vi "niFpgaHandshakeEmulationRefIn.vi"(0 "Name":variant, 5 "fourWireIn":bool, 7 "Data In":variant, 9 "Method":T1, 11 "Directly In SCTL":bool, 12 "Node Link":cluster{"VIRef":refnum<vi>, "UID":i32}) -> (6 "fourWireOut":bool, 8 "Data Out":variant)   [LabVIEW 2017]
uses:
  <vilib>/rvi/DataTransferAndStorage/Container/Common/niFpgaContainerMethod.ctl
  <vilib>/rvi/DataTransferAndStorage/Container/Common/niFpgaContainerMetaDataKey.ctl
  <instcachedir>/0/niFpgaHandshakeEmulation_5D8480C20A254BA19CE2ED138FC3D25A.lvgen/niFpgaHandshakeEmulation_5D8480C20A254BA19CE2ED138FC3D25A_000.vi
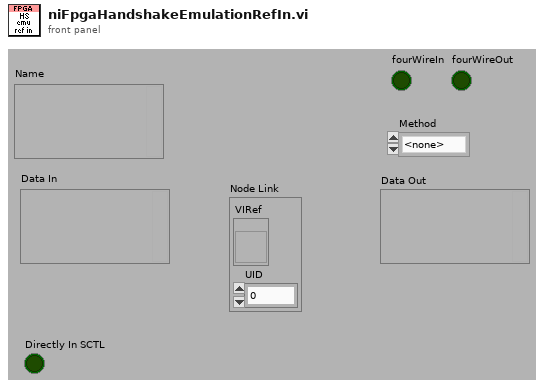
[diagram p1: front panel]
types:
  T1 = typedef "niFpgaContainerMethod.ctl" = enum16{"<none>", "write", "read", "clear", "getNumberOfElementsToWrite", "getNumberOfElementsToRead", "enable", "disable", "flushAndDisable", "getStreamState", "readA", "readB", "dramWrite", "dramWriteWithByteEnables", "dramRequestData", "dramRetrieveData", "readWithoutAcknowledge", "acknowledge", "writeUsingHandshaking", "readUsingHandshaking", "flush"}
  T2 = typedef "niFpgaContainerMetaDataKey.ctl" = enum16{"FPGA FIFO", "FPGA Memory", "FPGA Register", "FPGA Handshake"}
  T3 = typedef "niFpgaContainerState.ctl" = cluster{"displayName":string, "hardwareName":string, "dataType":T4, "elementTypeDescriptor":variant, "terminalTypeDescriptor":variant, "requestedNumberOfElements":u32, "memoryType":T5, "arbitrationForInterfaceA":T6, "numberOfElementsPerRead":u32, "arbitrationForInterfaceB":T6, "numberOfElementsPerWrite":u32, "VI_Defined":bool, "type":T7, "initializationParameters":T8, "disableOnOverflow/Underflow":bool, "interfaceConfiguration":T9, "controlLogic":T10, "actualNumberOfElements":u32, "dramSelection":string, "dramMaxOustandingRequests":i32, "dramIncludeByteEnables":bool, "dramGrantTime":u32, "fullEmulation":bool, "memoryInMultipleClockDomains":bool, "memoryLatency":T11}
  T4 = typedef "niFpgaDataTypeControl.ctl" = enum32{"Boolean", "I8", "I16", "I32", "I64", "U8", "U16", "U32", "U64", "FXP", "CustomControl", "SGL"}
  T5 = typedef "niFpgaContainerImplementationControl.ctl" = enum16{"Flip-Flops", "Look-Up Table", "Block Memory", "DRAM"}
  T6 = typedef "niFpgaContainerArbitrationOptionsControl.ctl" = enum16{"Always Arbitrate", "Arbitrate if Multiple Requestors Only", "Never Arbitrate"}
  T7 = typedef "niFpgaTransferTypeControl.ctl" = enum16{"Target-Scoped", "Host to Target - DMA", "Target to Host - DMA", "Peer to Peer Reader", "Peer to Peer Writer", "Bidirectional"}
  T8 = typedef "niFpgaContainerInitializationParameters.ctl" = cluster{"initialized":bool, "VI_Path":path, "initialData":variant}
  T9 = typedef "niFpgaMemoryInterfaceConfiguration.ctl" = enum16{"Read A-Write B", "Read A-Read B"}
  T10 = typedef "niFpgaFifoControlLogicControl.ctl" = enum16{"Slice Fabric", "Target Optimal", "Built-in"}
  T11 = typedef "niFpgaContainerMemoryLatencyControl.ctl" = u16
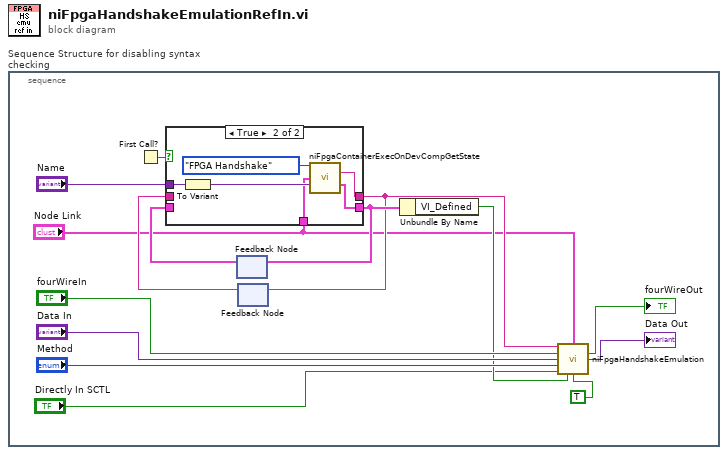
[diagram p0: block diagram]
diagram:
  n1 = stacked-sequence "Sequence Structure for disabling syntax checking" {
    frame #0 {
      n2 = First Call?() -> (First Call?: T/F=w9:bool)
      n3 = feedback #1() -> (w7:T3)  [unwired: 1 out]
      n4 = feedback #2() -> (w6:string)  [unwired: 1 out]
      n5 = case shown="True" w9 {
        tunnel: "Name" -> [_ w23]
        tunnel: [w17 w19] -> w8
        tunnel: w7 -> [w17 _]
        tunnel: [w16 w20] -> w5
        tunnel: w6 -> [w16 _]
        tunnel: "Node Link" -> [_ w18]
        frame False {
        }
        frame True {
          n6 = To Variant(anything=w23) -> (Variant=w22:variant)
          n7 = call <vilib>:"niFpgaContainerExecOnDevCompGetState.vi"("containerMetaDataKey"=niFpgaContainerMetaDataKey."FPGA Handshake", "Node Link"=w18, "name"=w22) -> ("Unique  Name"=w20:string, "containerState"=w19:T3)  [unwired: 3 in, 8 out]
        }
      }
      n8 = feedback-in #1(w8) -> ()
      n9 = feedback-in #2(w5) -> ()
      n10 = Unbundle By Name(w8) -> ("VI_Defined"=w3:bool)
      n11 = call-generic <vilib>:"niFpgaHandshakeEmulation.vi"("name"=w5, "Node Link"="Node Link", "fourWireIn"="fourWireIn", "data in"="Data In", "Method"="Method", "Directly In SCTL"="Directly In SCTL", "Local? (F)"=w3, "Ref In wired (F)"=TRUE ("ref in wired")) -> ("fourWireOut"=→"fourWireOut":bool, "data out"=→"Data Out":variant)  [unwired: 6 in]
    }
  }
